vi "Replace Meta Inforamtion.vi"(6 "bookmark as key(T)\n/content as key(F)":bool=TRUE, 8 "error in (no error)":errorcluster, 10 "bookmark name":string, 11 "Word_Report in":refnum<class "Word_Report.lvclass">) -> (0 "error out":errorcluster, 3 "Word_Report out":refnum<class "Word_Report.lvclass">)   [LabVIEW 2018]
uses:
  Word_Report.lvclass
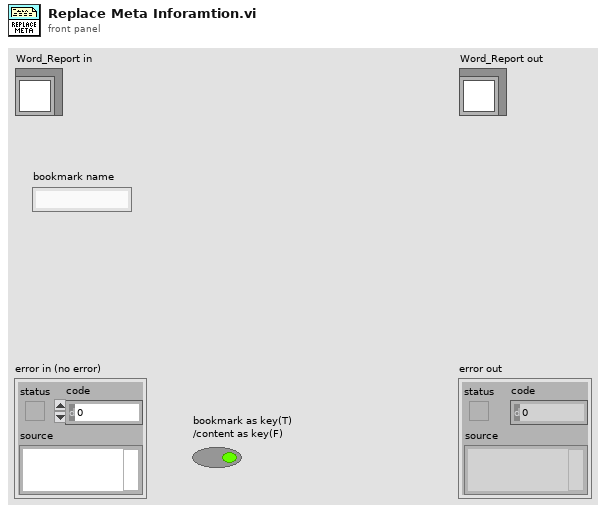
[diagram p1: front panel]
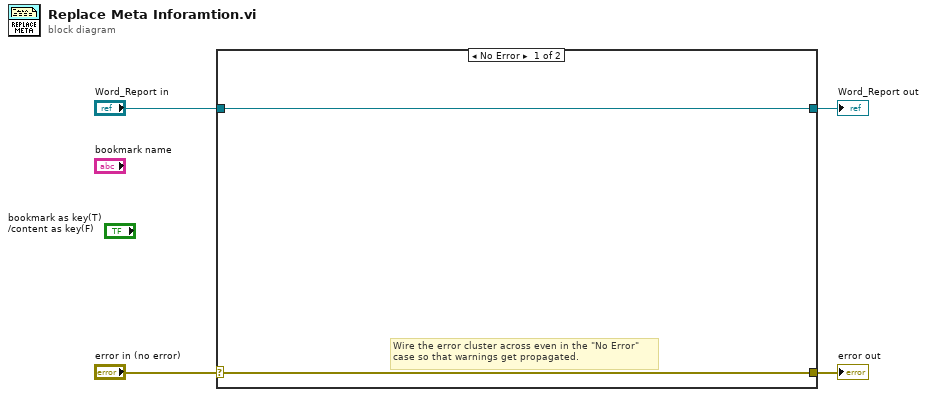
[diagram p0: block diagram]
diagram:
  n1 = case shown="No Error" "error in (no error)" {
    selector: "error in (no error)" -> [w5 w8]
    tunnel: [w5 w8] -> w3
    tunnel: [w6 w7] -> w1
    tunnel: "Word_Report in" -> [w6 w7]
    frame No Error {
      # "Wire the error cluster across even in the \"No Error\"\ncase so that warnings get propagated."
    }
    frame Error {
    }
  }
  "error out" <- w3
  "Word_Report out" <- w1
